vi "FGEN Post Sub Steps.vi"(9 "Socket Index":i16, 10 "FGEN_IN":T1={"Enable Output"=FALSE, "Amplitude (Vp-p) "=1.0, "Frequency (Hz)"=1000000.0, "DC Offset (V)"=0.0, "Start Phase"=0.0, "Standard Waveform"=0, "FGEN Operation"=enum."Configure", "Active Channel"=""} {"Standard Waveform" scale=0.0..6.0; "DC Offset (V)" min=-6.0 max=6.0 scale=-6.0..6.0 scale format="%_1p"; "Frequency (Hz)" min=9000.0 max=100000000.0 scale=0.0..100000000.0 scale format="%_1p"; "Amplitude (Vp-p)" min=0.0 max=12.0 scale=0.0..12.0 scale format="%.1f"}, 11 "Sequence Context In":refnum<k7>) -> (0 "error out":errorcluster, 2 "FGEN_Out":T1={"Enable Output"=FALSE, "Amplitude (Vp-p) "=1.0, "Frequency (Hz)"=1000000.0, "DC Offset (V)"=0.0, "Start Phase"=0.0, "Standard Waveform"=0, "FGEN Operation"=enum."Configure", "Active Channel"=""} {"Standard Waveform" scale=0.0..6.0; "DC Offset (V)" min=-6.0 max=6.0 scale=-6.0..6.0 scale format="%_1p"; "Frequency (Hz)" min=9000.0 max=100000000.0 scale=0.0..100000000.0 scale format="%_1p"; "Amplitude (Vp-p)" min=0.0 max=12.0 scale=0.0..12.0 scale format="%.1f"}, 3 "Report Text":string)   [LabVIEW 2023, in "LTT_TeststandSteptypes.lvlib"]
uses:
  LTT_TeststandSteptypes.lvlib
  Control/FGEN Data.ctl
  HardwareAbstractionLayer_LVOOP/Function Generator/Function Generator.lvclass
  HardwareAbstractionLayer_LVOOP/Database/Database.lvclass
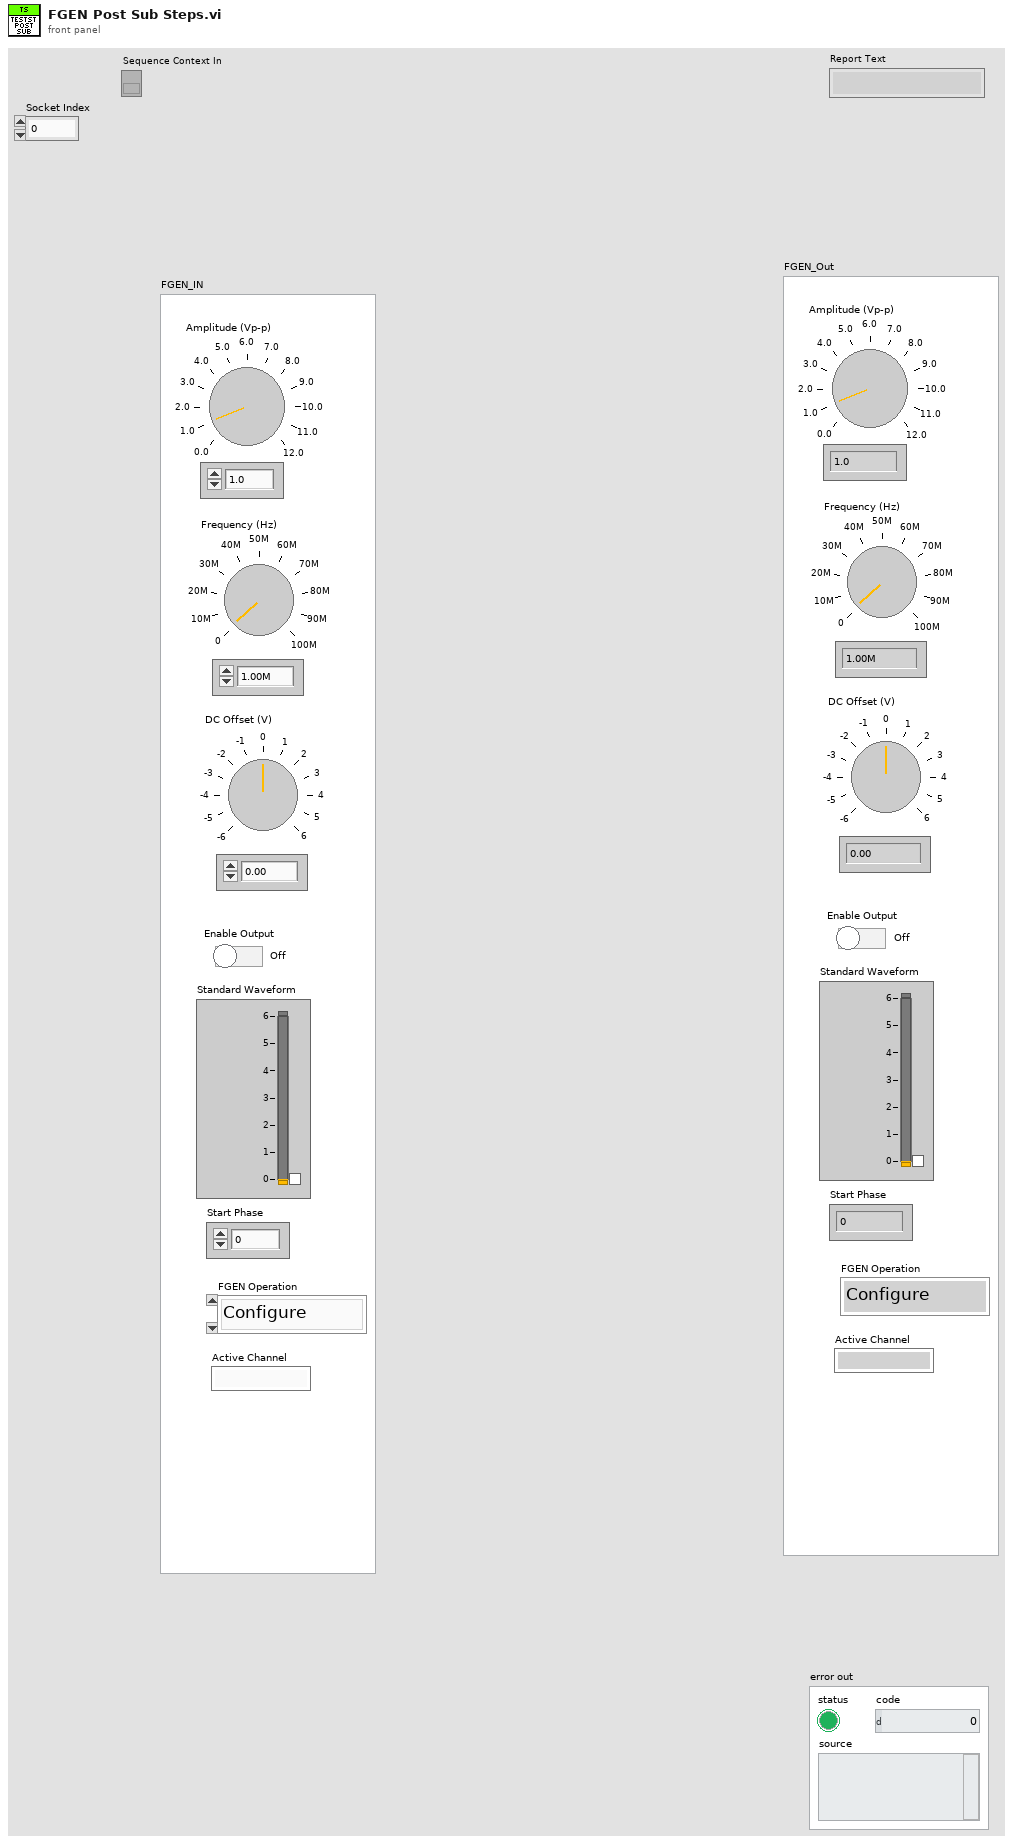
[diagram p1: front panel]
types:
  T1 = typedef "LTT_TeststandSteptypes.lvlib/FGEN Data.ctl" = cluster{"Enable Output":bool, "Amplitude (Vp-p) ":dbl, "Frequency (Hz)":dbl, "DC Offset (V)":dbl, "Start Phase":dbl, "Standard Waveform":u16, "FGEN Operation":enum32{"Init", "Self Test", "Configure Channel", "Configure", "Start", "Stop", "Measure", "Close"}, "Active Channel":string}
  T2 = enum32{"Init", "Self Test", "Configure Channel", "Configure", "Start", "Stop", "Measure", "Close"}
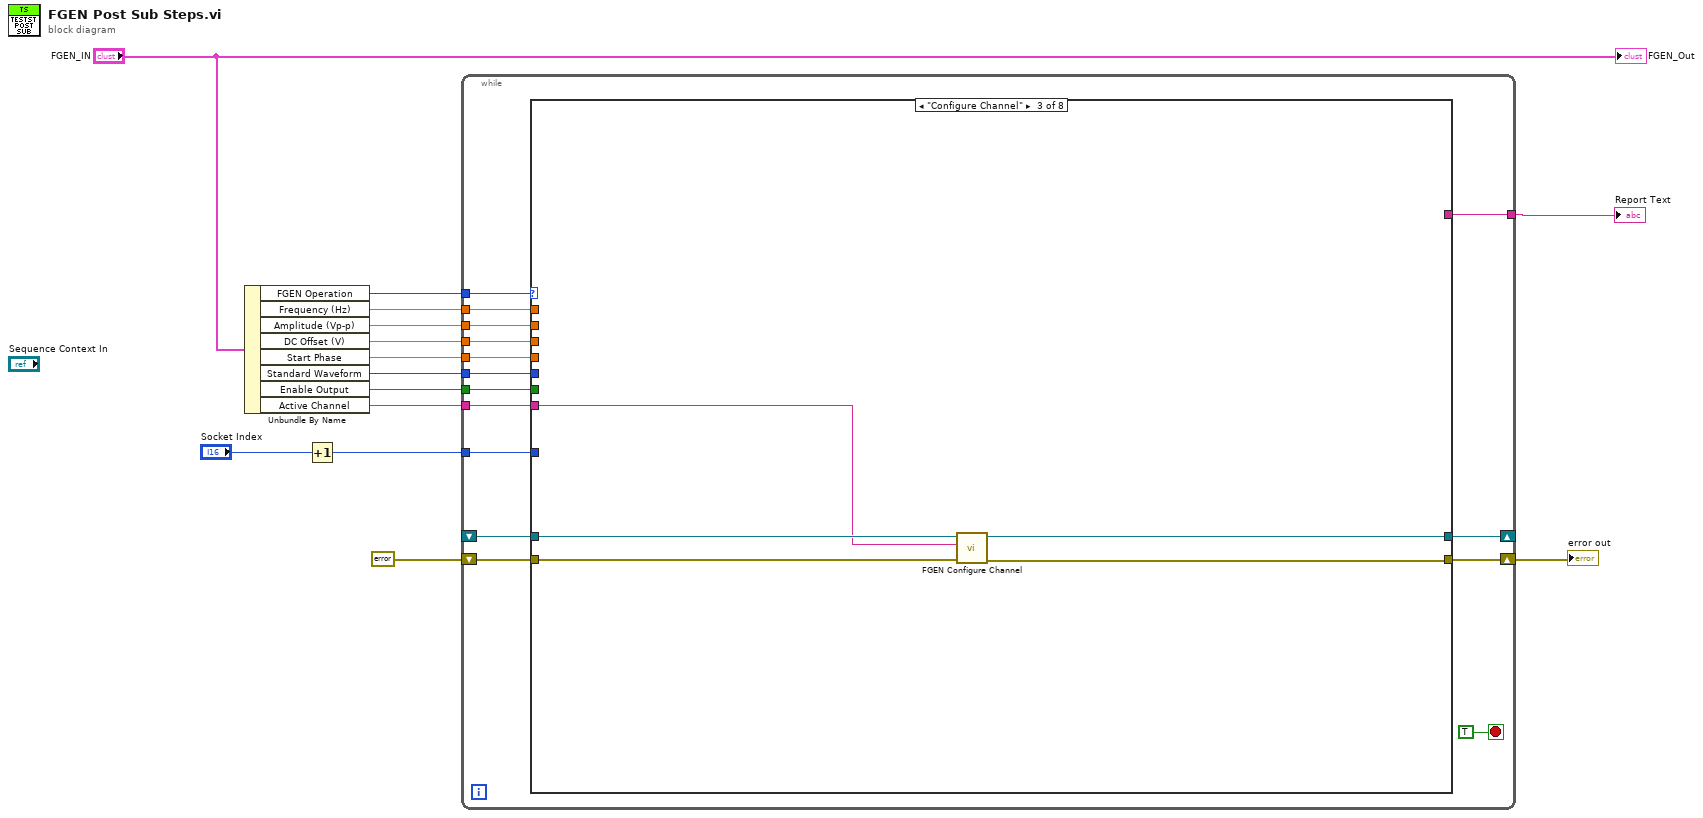
[diagram p0: block diagram]
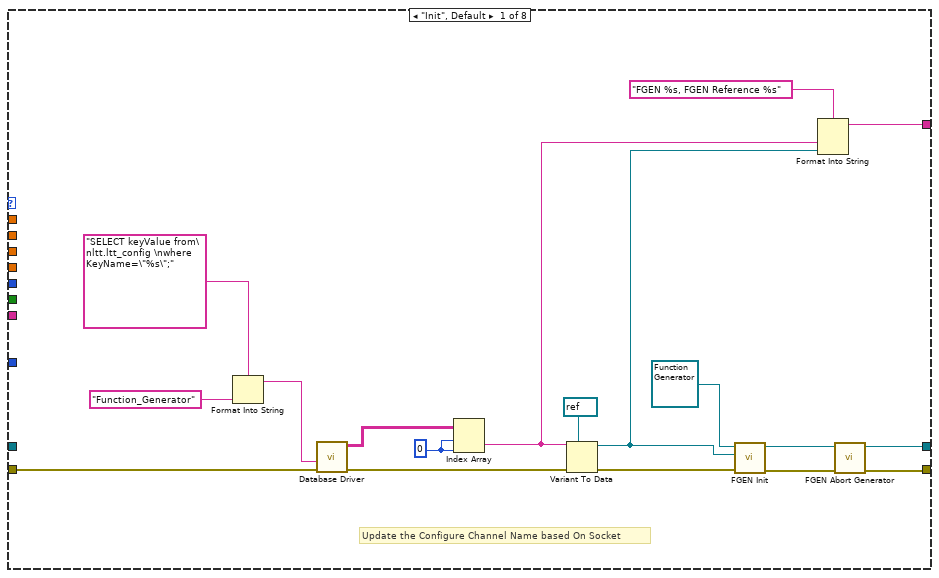
[diagram p2: hidden frame]
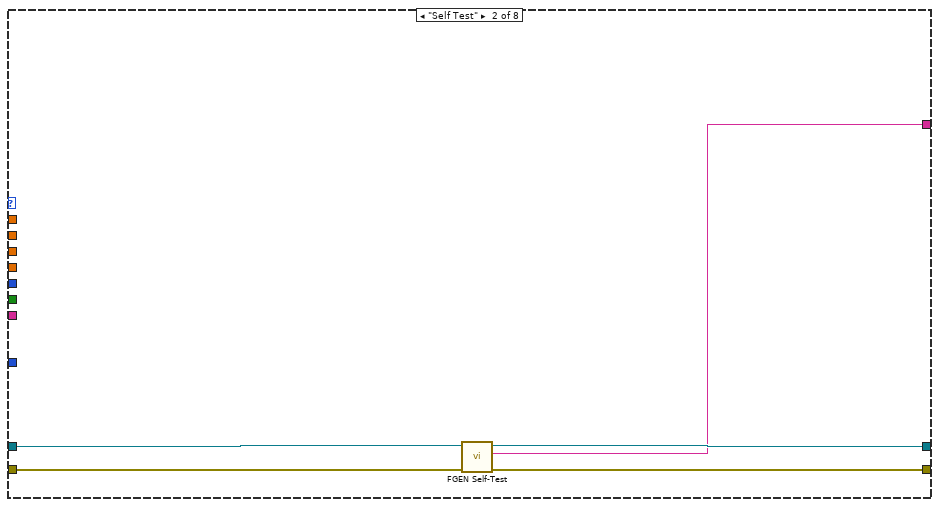
[diagram p3: hidden frame]
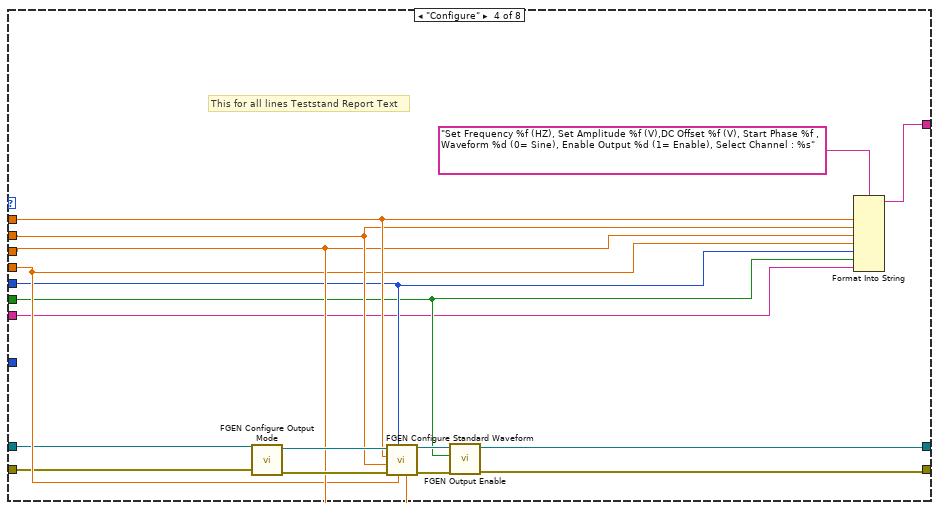
[diagram p4: hidden frame]
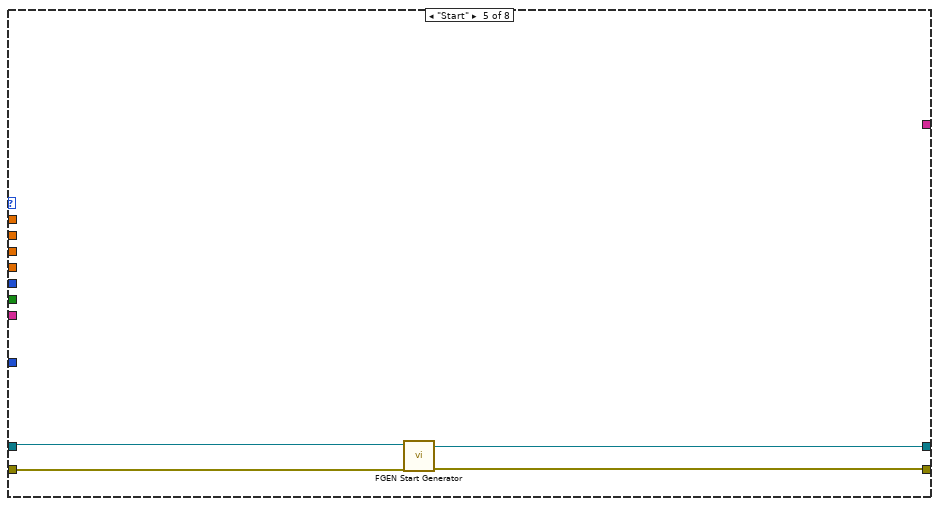
[diagram p5: hidden frame]
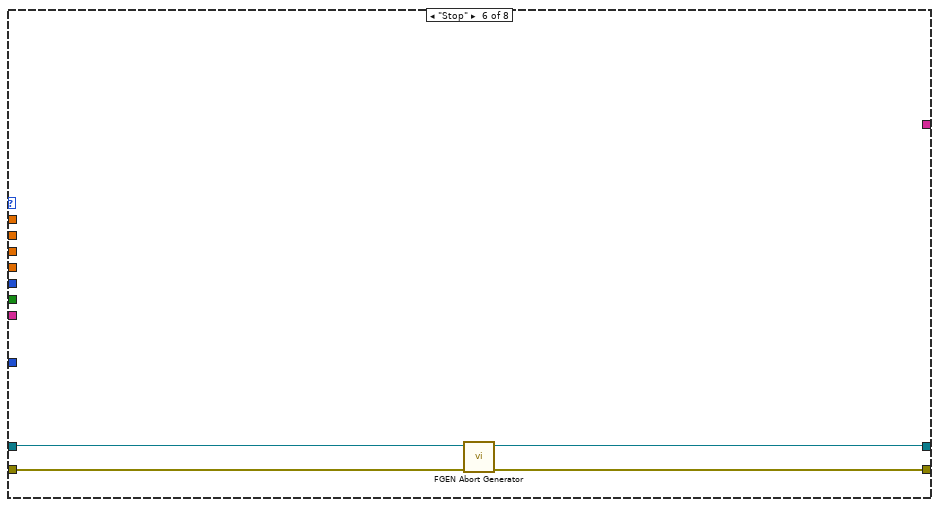
[diagram p6: hidden frame]
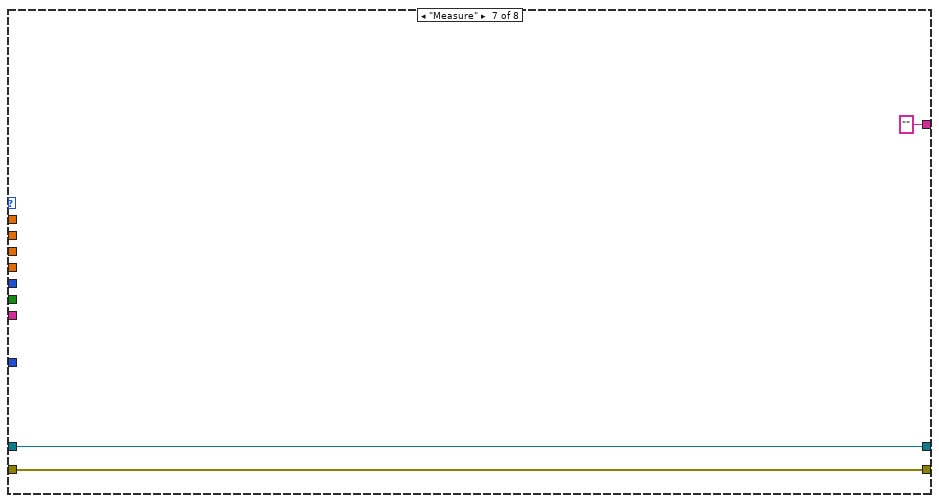
[diagram p7: hidden frame]
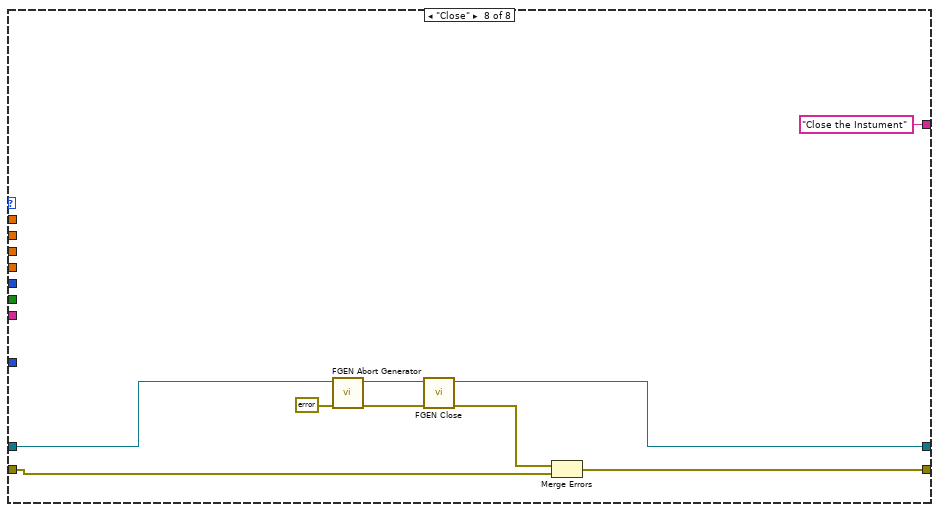
[diagram p8: hidden frame]
diagram:
  n1 = Unbundle By Name("FGEN_IN") -> ("FGEN Operation"=w10:T2, "Frequency (Hz)"=w9:dbl, "Amplitude (Vp-p)"=w8:dbl, "DC Offset (V)"=w7:dbl, "Start Phase"=w6:dbl, "Standard Waveform"=w5:u16, "Enable Output"=w4:bool, "Active Channel"=w1:string)
  n2 = Increment(x="Socket Index") -> (x+1=w13:i16)
  n3 = while {
    tunnel: w10 -> [w28]
    shift-right: [w26] -> w2
    shift-left: errorcluster {"status"=FALSE, "code"=0, "source"=""} ("error in") -> [w27]
    tunnel: w13 -> [w25]
    tunnel: [w24] -> w3
    shift-right: [w23] -> _
    shift-left: _ -> [w22]
    tunnel: w9 -> [w21]
    tunnel: w8 -> [w20]
    tunnel: w7 -> [w19]
    tunnel: w6 -> [w18]
    tunnel: w5 -> [w17]
    tunnel: w4 -> [w16]
    tunnel: w1 -> [w15]
    stop <- TRUE stop-if-true
    n4 = case shown="\"Configure Channel\"" w28 {
      tunnel: w27 -> [w44 w51 w57 w58 w77 w81 w85 w88]
      tunnel: [w31 w50 w56 w67 w76 w80 w85 w93] -> w26
      tunnel: w25 -> [_ _ _ _ _ _ _ _]
      tunnel: [w42 w48 _ w73 _ _ "" ("Self-Test Result Message") "Close the Instument" ("Self-Test Result Message")] -> w24
      tunnel: [w33 w49 w54 w68 w75 w79 w83 w87] -> w23
      tunnel: w22 -> [_ w52 w55 w59 w78 w82 w83 w92]
      tunnel: w21 -> [_ _ _ w66 _ _ _ _]
      tunnel: w20 -> [_ _ _ w65 _ _ _ _]
      tunnel: w19 -> [_ _ _ w64 _ _ _ _]
      tunnel: w18 -> [_ _ _ w63 _ _ _ _]
      tunnel: w17 -> [_ _ _ w62 _ _ _ _]
      tunnel: w16 -> [_ _ _ w61 _ _ _ _]
      tunnel: w15 -> [_ _ w53 w60 _ _ _ _]
      frame "Init", Default {
        w47 = 0 ("index (row)")
        # "Update the Configure Channel Name based On Socket"
        n5 = Format Into String(format string="SELECT keyValue from\nltt.ltt_config \nwhere KeyName=\"%s\";", "Function_Generator" ("input 1")) -> (resulting string=w46:string)  [unwired: 2 in, 1 out]
        n6 = call "Database Driver.vi"("error in"=w44, "SQL query"=w46) -> ("error out"=w43:errorcluster, "data"=w45:string[][])  [unwired: 6 in, 2 out]
        n7 = Index Array(array=w45, index (row)=w47, index (col)=w47) -> (element=w38:string)
        n8 = Variant To Data(error in=w43, type=refnum<k15> refnum ("Resource Name"), Variant=w38) -> (data=w30:refnum<k15>, error out=w36:errorcluster)
        n9 = call-dynamic "FGEN Init.vi"("error in (no error)"=w36, "Resource Name"=w30, "Function Generator in"=refnum<class "Function Generator.lvclass"> refnum ("HardwareAbstractionLayer_LVOOP.lvlib:Function Generator.lvclass")) -> ("error out"=w32:errorcluster, "Function Generator out"=w34:refnum<class "Function Generator.lvclass">)  [unwired: 7 in]
        n10 = Format Into String(format string="FGEN %s, FGEN Reference %s", w38, w30) -> (resulting string=w42:string)  [unwired: 2 in, 1 out]
        n11 = call-dynamic "FGEN Abort Generator.vi"("error in (no error)"=w32, "Function Generator in"=w34) -> ("error out"=w31:errorcluster, "Function Generator out"=w33:refnum<class "Function Generator.lvclass">)  [unwired: 8 in]
      }
      frame "Self Test" {
        n12 = call-dynamic "FGEN Self-Test.vi"("error in (no error)"=w51, "Function Generator in"=w52) -> ("error out"=w50:errorcluster, "Report Text"=w48:string, "Function Generator out"=w49:refnum<class "Function Generator.lvclass">)  [unwired: 7 in]
      }
      frame "Configure Channel" {
        n13 = call-dynamic "FGEN Configure Channel.vi"("error in (no error)"=w57, "Active Channel"=w53, "Function Generator in"=w55) -> ("error out"=w56:errorcluster, "Function Generator out"=w54:refnum<class "Function Generator.lvclass">)  [unwired: 7 in]
      }
      frame "Configure" {
        # "This for all lines Teststand Report Text"
        n14 = call-dynamic "FGEN Configure Output Mode.vi"("error in (no error)"=w58, "Function Generator in"=w59) -> ("error out"=w71:errorcluster, "Function Generator out"=w72:refnum<class "Function Generator.lvclass">)  [unwired: 8 in]
        n15 = call-dynamic "FGEN Configure Standard Waveform.vi"("DC Offset (V)"=w64, "Start Phase"=w63, "Standard Waveform"=w62, "error in (no error)"=w71, "Amplitude (Vp-p)"=w65, "Frequency (Hz)"=w66, "Function Generator in"=w72) -> ("error out"=w70:errorcluster, "Function Generator out"=w69:refnum<class "Function Generator.lvclass">)  [unwired: 3 in]
        n16 = call-dynamic "FGEN Output Enable.vi"("error in (no error)"=w70, "Output Enable (default: True)"=w61, "Function Generator in"=w69) -> ("error out"=w67:errorcluster, "Function Generator out"=w68:refnum<class "Function Generator.lvclass">)  [unwired: 7 in]
        n17 = Format Into String(format string="Set Frequency %f (HZ), Set Amplitude %f (V),DC Offset %f (V), Start Phase %f , Waveform %d (0= Sine), Enable Output %d (1= Enable), Select Channel : %s", w66, w65, w64, w63, w62, w61, w60) -> (resulting string=w73:string)  [unwired: 2 in, 1 out]
      }
      frame "Start" {
        n18 = call-dynamic "FGEN Start Generator.vi"("error in (no error)"=w77, "Function Generator in"=w78) -> ("error out"=w76:errorcluster, "Function Generator out"=w75:refnum<class "Function Generator.lvclass">)  [unwired: 8 in]
      }
      frame "Stop" {
        n19 = call-dynamic "FGEN Abort Generator.vi"("error in (no error)"=w81, "Function Generator in"=w82) -> ("error out"=w80:errorcluster, "Function Generator out"=w79:refnum<class "Function Generator.lvclass">)  [unwired: 8 in]
      }
      frame "Measure" {
      }
      frame "Close" {
        n20 = call-dynamic "FGEN Abort Generator.vi"("error in (no error)"=errorcluster {"status"=FALSE, "code"=0, "source"=""}, "Function Generator in"=w92) -> ("error out"=w91:errorcluster, "Function Generator out"=w90:refnum<class "Function Generator.lvclass">)  [unwired: 8 in]
        n21 = call-dynamic "FGEN Close.vi"("error in (no error)"=w91, "Function Generator in"=w90) -> ("error out"=w89:errorcluster, "Function Generator out"=w87:refnum<class "Function Generator.lvclass">)  [unwired: 8 in]
        n22 = Merge Errors(w89, w88) -> (w93:errorcluster)
      }
    }
  }
  "Report Text" <- w3
  "error out" <- w2
  "FGEN_Out" <- "FGEN_IN"
